vi "GUI_kHz_Control_Center.vi"() -> ()   [LabVIEW 2020]
uses:
  Shared/GUI_Template/GUI_master/tcp_new_data_event.ctl
  Shared/GUI_Template/GUI_master/tcp new data cluster.ctl
panel:
  in  "BASE PATH":path=path "Z:/software/control-all-loasis/kHz LPA/Active Version"
  in  "stop":bool=TRUE
  in  "Tab Control":enum32{"Devices", "Parameters"}(tab)=enum."Parameters"
  out "tcp data event":T1
  out "error IO 2":errorcluster
  in  "GUIdevice 2":string="kHz_1Wire"
  in  "GUIdevice 1":string="kHz_Alicat"
  out "GUIdevice 0":string="kHz_Alicat"
  in  "GUIdevice 3":string="kHz_Hexapod_Target"
  in  "GUIdevice 4":string="kHz_DG645_ShotControl"
  in  "GUIdevice 5":string="kHz_Zaber_Compressor"
  in  "Position.Ch1::5":i32 caption="Ch1" min=0 max=250000 step=1
  in  "Google Drive":bool
  in  "MasterControl":bool caption="PicoL GUI"
  in  "LVStarter":bool caption="PicoL GUI"
  in  "GEECSplot":bool caption="PicoL GUI"
  in  "AddColumns":bool caption="PicoL GUI"
  in  "DB Editor":bool caption="PicoL GUI"
  in  "Exp Editor":bool caption="PicoL GUI"
  in  "HTT Interactive":bool caption="PicoL GUI"
  in  "RemoteDesktop":bool caption="PicoL GUI"
  in  "Search Log":bool caption="PicoL GUI"
  in  "LogTable":bool
  in  "New Google\nExpLog for new day?":bool=TRUE
  in  "LogEpilog":bool caption="LogTable"
  in  "Scan":T2(ring)
  in  "Create Log":bool caption="LogTable"
  in  "Position.Channel 1::2":T3(ring) caption="XH1"
  in  "Position.Channel 2::2":T3(ring) caption="XH2"
  in  "Position.Channel 3::2":T3(ring) caption="XH3"
  in  "Position.Channel 4::2":T3(ring) caption="XH4"
  in  "Position.Channel 5::2":T3(ring) caption="d-scan wedge"
  in  "Position.Channel 6::2":T3(ring) caption="EC wedge"
  in  "Position.Channel 8::2":T3(ring) caption="ND6+"
  in  "Position.Channel 7::2":T3(ring) caption="ExitMode wedge"
  in  "Pressure.device 1::1":dbl caption="Target Pressure" min=0.0 max=100.0
  in  "Pressure.device 2::1":dbl caption="Fiber Pressure" min=-14.7 max=500.0
  in  "xpos::3":dbl=-18.95 caption="x" min=-22.5 max=22.5 step=0.01 format="%.5f"
  in  "zpos::3":dbl=-0.7 caption="z" min=-10.0 max=10.0 step=0.01 format="%.5f"
  in  "ypos::3":dbl=10.7 caption="y" min=-22.5 max=22.5 step=0.01 format="%.5f"
  in  "uangle::3":dbl caption="u" min=-7.5 max=7.5 step=0.01 format="%.5f"
  in  "vangle::3":dbl=0.0007 caption="v" min=-7.5 max=7.5 step=0.01 format="%.5f"
  in  "wangle::3":dbl=-0.0001 caption="w" min=-7.5 max=7.5 step=0.01 format="%.5f"
  in  "fire::4":string
  # "kHz control center"
  # "Hexapod"
  # "1-wire flippers"
  # "Laser"
  # "\"+x\" is towards laser table\n\"+y\" is towards OAP\n\"+z\" is up"
  # "Tobi's LogMaker"
  # "Alicat"
  # "New\nScan\nTable"
  # "Compressor"
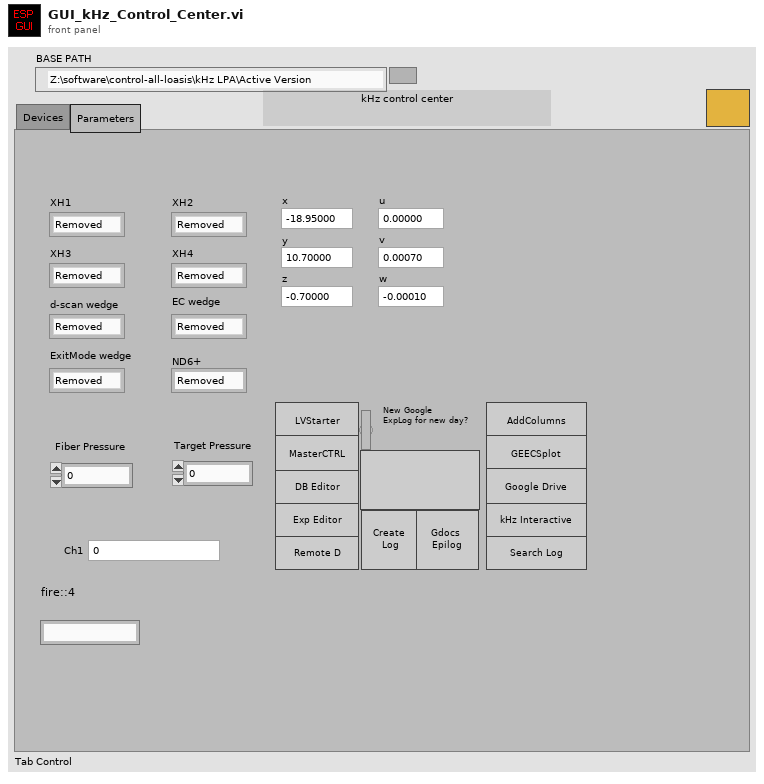
[diagram p1: front panel]
types:
  T1 = typedef "tcp_new_data_event.ctl" = refnum<user-event>
  T2 = enum16{"0", "1", "2", "3", "4", "5", "6", "7", "8", "9", "10", "11", "12", "13", "14", "15", "16", "17", "18", "19", "20", "21", "22", "23", "24", "25", "26", "27", "28", "29", "30", "31", "32", "33", "34", "35", "36", "37", "38", "39", "40", "41", "42", "43", "44", "45", "46", "47", "48", "49", "50", "51", "52", "53", "54", "55", "56", "57", "58", "59", "60", "61", "62", "63", "64", "65", "66", "67", "68", "69", "70", "71", "72", "73", "74", "75", "76", "77", "78", "79", "81", "82", "83", "84", "85", "86", "87", "88", "89", "90", "91", "92", "93", "94", "95", "96", "97", "98", "99", ""}
  T3 = enum16{"Removed", "Inserted", "Unknown", "Moving"}
  T4 = typedef "tcp new data cluster.ctl" = cluster{"EventEnum":enum16{"new data", "connection status update"}, "Device name":string}
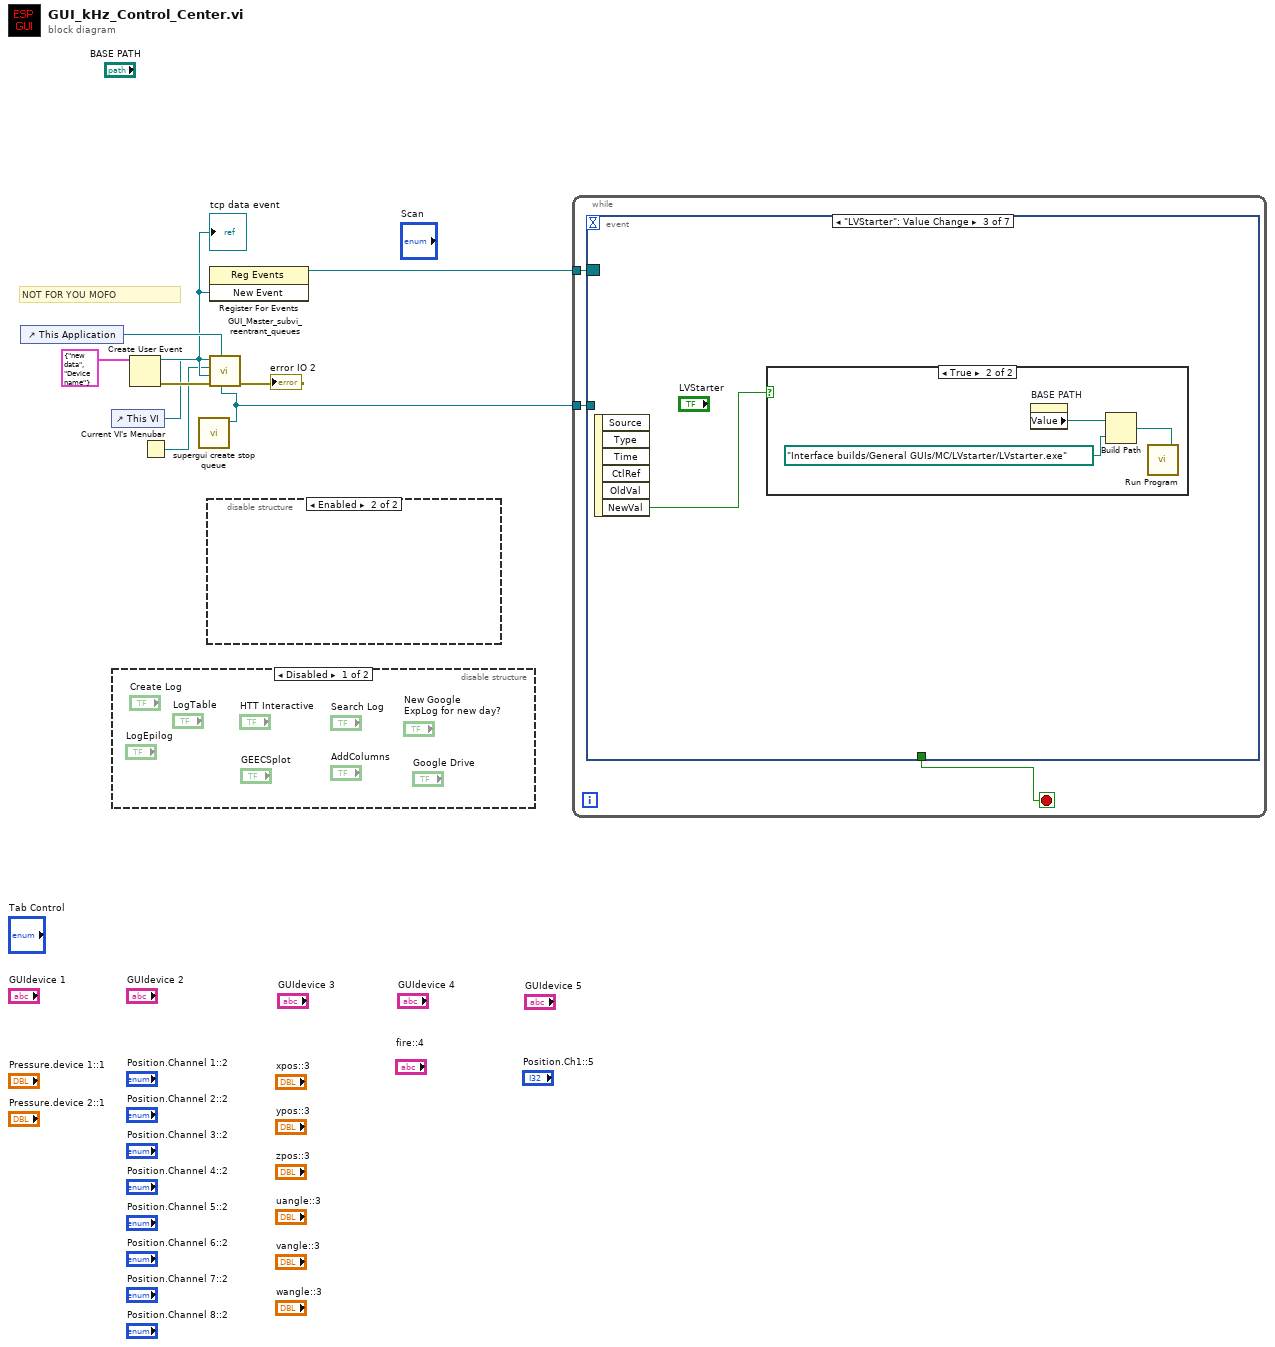
[diagram p0: block diagram]
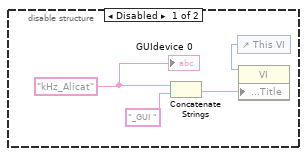
[diagram p3: hidden frame]
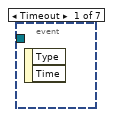
[diagram p4: hidden frame]
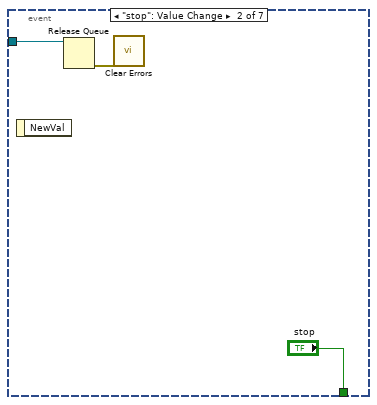
[diagram p5: hidden frame]
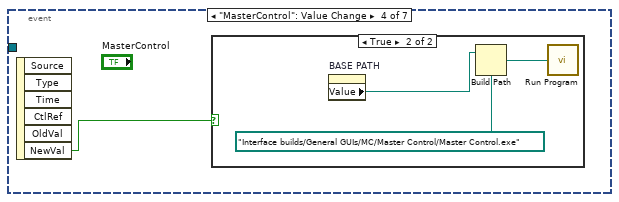
[diagram p7: hidden frame]
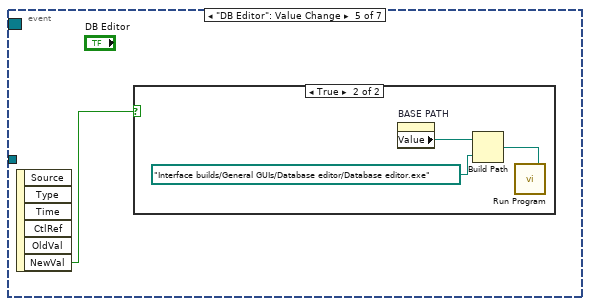
[diagram p9: hidden frame]
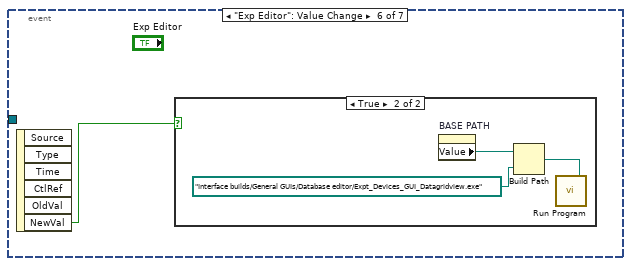
[diagram p11: hidden frame]
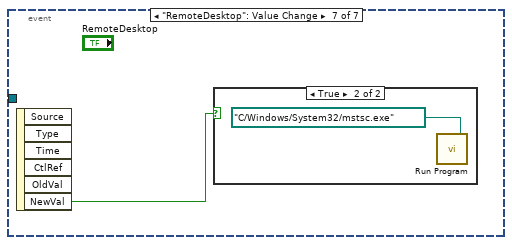
[diagram p13: hidden frame]
diagram:
  # "NOT FOR YOU MOFO"
  n1 = control-ref of="This Application"() -> (w9:refnum<vi>)
  n2 = control-ref of="This VI"() -> (w4:refnum<vi>)
  n3 = disable-structure shown="Disabled" {
    frame Disabled {
    }
    frame Enabled {
    }
  }
  n4 = Create User Event(user event datatype=T4 {"EventEnum"=enum."new data", "Device name"="Device name"} ("New Event")) -> (user event=w8:refnum<user-event>, error out=w7:errorcluster)  [unwired: 1 in]
  "tcp data event" <- w8
  n5 = Current VI's Menubar() -> (w5:refnum<k9>)
  n6 = call "supergui create stop queue.vi"() -> ("STOP Queue out"=w1:refnum<queue>)  [unwired: 11 in]
  n7 = disable-structure shown="Enabled" {
    frame Disabled {
      w10 = "kHz_Alicat" ("GUIdevice 1")
      n8 = Concatenate Strings(w10, "_GUI ") -> (w12:string)
      n9 = control-ref of="This VI"() -> (w13:refnum<vi>)
      n10 = property class="VI"(reference=w13, "Front Panel.Title"=w12) -> ()  [unwired: 1 in, 2 out]
      "GUIdevice 0" <- w10
    }
    frame Enabled {
    }
  }
  n11 = register-events(w8) -> (reference out=w2:refnum<event-registration>)  [unwired: 2 in, 1 out]
  n12 = call "GUI_Master_subvi_reentrant_queues.vi"("STOP Queue in"=w1, "This Application"=w9, "error in (no error)"=w7, "tcp data event"=w8, "Caller menu reference"=w5, "Caller VI ref"=w4) -> ("error out"=→"error IO 2":errorcluster)  [unwired: 5 in]
  n13 = while {
    tunnel: w2 -> [w16]
    tunnel: w1 -> [w14]
    stop <- w15 stop-if-true
    n14 = event shown="[2] \"LVStarter\": Value Change" {
      selector: w16 -> [_ _ _ _ _ _ _]
      dyn-events: _ -> [_ _ _ _ _ _ _]
      timeout: _ -> [_ _ _ _ _ _ _]
      tunnel: [_ "stop" _ _ _ _ _] -> w15
      tunnel: w14 -> [_ w18 _ _ _ _ _]
      event Timeout {
        n15 = event-data() -> ()  [unwired: 1 in, 2 out]
      }
      event "stop": Value Change {
        n16 = event-data() -> ()  [unwired: 1 in, 1 out]
        n17 = Release Queue(queue=w18) -> (error out=w17:errorcluster)  [unwired: 2 in, 2 out]
        n18 = call <vilib>:"Clear Errors.vi"("error in (no error)"=w17) -> ()  [unwired: 5 in, 2 out]
      }
      event "LVStarter": Value Change {
        n19 = event-data() -> ("NewVal"=w20:bool)  [unwired: 1 in, 5 out]
        n20 = case shown="True" w20 {
          frame False {
          }
          frame True {
            n21 = property on="BASE PATH" class="Path"() -> ("Value"=w21:path)  [unwired: 2 in, 2 out]
            n22 = Build Path(base path=w21, name or relative path=path "Interface builds/General GUIs/MC/LVstarter/LVstarter.exe") -> (appended path=w23:path)
            n23 = call "Run Program.vi"("Program Path"=w23) -> ()  [unwired: 1 in]
          }
        }
      }
      event "MasterControl": Value Change {
        n24 = event-data() -> ("NewVal"=w24:bool)  [unwired: 1 in, 5 out]
        n25 = case shown="True" w24 {
          frame False {
          }
          frame True {
            n26 = property on="BASE PATH" class="Path"() -> ("Value"=w25:path)  [unwired: 2 in, 2 out]
            n27 = Build Path(base path=w25, name or relative path=path "Interface builds/General GUIs/MC/Master Control/Master Control.exe") -> (appended path=w27:path)
            n28 = call "Run Program.vi"("Program Path"=w27) -> ()  [unwired: 1 in]
          }
        }
      }
      event "DB Editor": Value Change {
        n29 = event-data() -> ("NewVal"=w28:bool)  [unwired: 1 in, 5 out]
        n30 = case shown="True" w28 {
          frame False {
          }
          frame True {
            n31 = property on="BASE PATH" class="Path"() -> ("Value"=w29:path)  [unwired: 2 in, 2 out]
            n32 = Build Path(base path=w29, name or relative path=path "Interface builds/General GUIs/Database editor/Database editor.exe") -> (appended path=w31:path)
            n33 = call "Run Program.vi"("Program Path"=w31) -> ()  [unwired: 1 in]
          }
        }
      }
      event "Exp Editor": Value Change {
        n34 = event-data() -> ("NewVal"=w32:bool)  [unwired: 1 in, 5 out]
        n35 = case shown="True" w32 {
          frame False {
          }
          frame True {
            n36 = property on="BASE PATH" class="Path"() -> ("Value"=w33:path)  [unwired: 2 in, 2 out]
            n37 = Build Path(base path=w33, name or relative path=path "Interface builds/General GUIs/Database editor/Expt_Devices_GUI_Datagridview.exe") -> (appended path=w35:path)
            n38 = call "Run Program.vi"("Program Path"=w35) -> ()  [unwired: 1 in]
          }
        }
      }
      event "RemoteDesktop": Value Change {
        n39 = event-data() -> ("NewVal"=w36:bool)  [unwired: 1 in, 5 out]
        n40 = case shown="True" w36 {
          frame False {
          }
          frame True {
            n41 = call "Run Program.vi"("Program Path"=path "C:/Windows/System32/mstsc.exe") -> ()  [unwired: 1 in]
          }
        }
      }
    }
  }
